vi "Main.vi"(0 "Temperature":dbl, 5 "Pressure":dbl, 7 "String 1":string, 9 "String 2":string, 11 "Error in":errorcluster) -> (15 "Error out":errorcluster)   [LabVIEW 2020, in "Menu.lvlib"]
doc: "This VI is just used to implement the run time menu feature where controls are enabled and disabled with the help of run time menu"
uses:
  Menu.lvlib
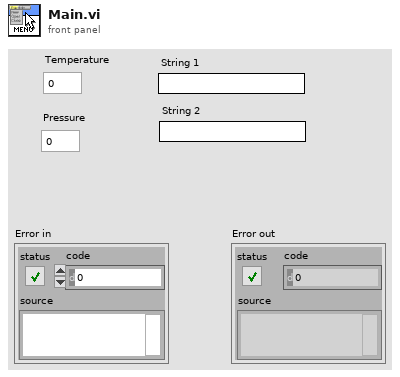
[diagram p1: front panel]
types:
  T1 = enum8{"Enabled", "Disabled", "Disabled and Grayed Out"}
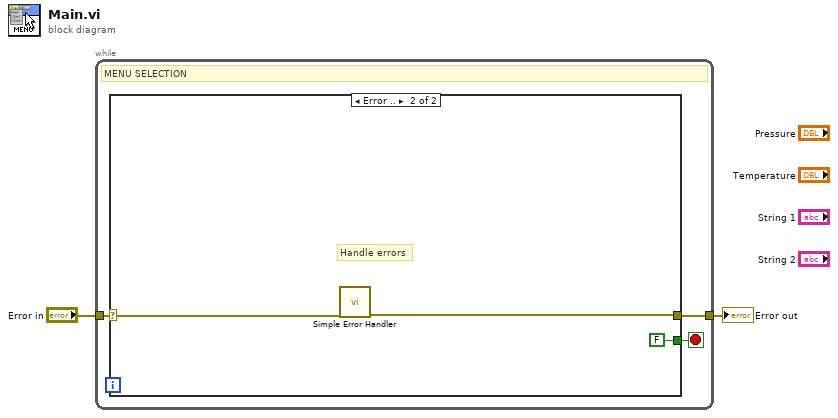
[diagram p0: block diagram]
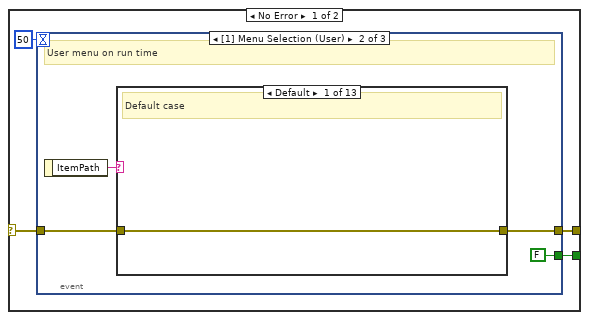
[diagram p2: hidden frame]
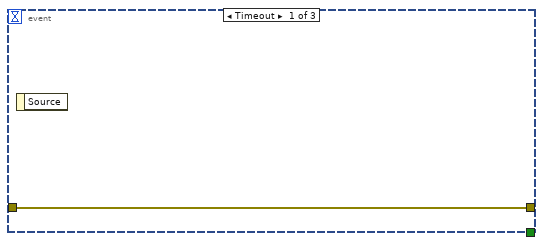
[diagram p3: hidden frame]
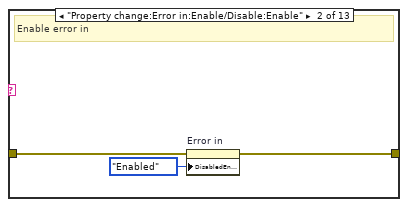
[diagram p4: hidden frame]
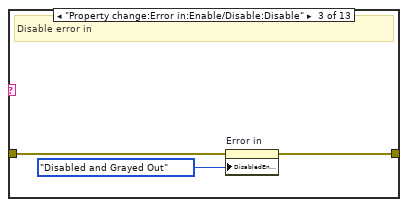
[diagram p5: hidden frame]
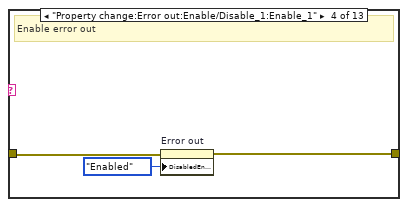
[diagram p6: hidden frame]
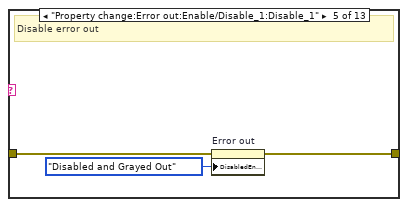
[diagram p7: hidden frame]
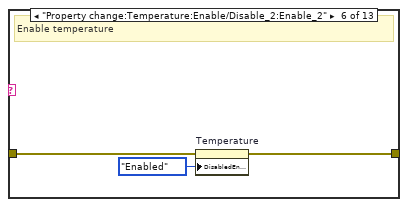
[diagram p8: hidden frame]
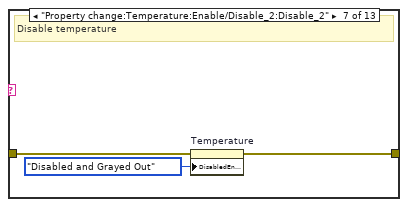
[diagram p9: hidden frame]
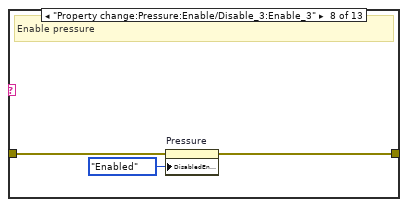
[diagram p10: hidden frame]
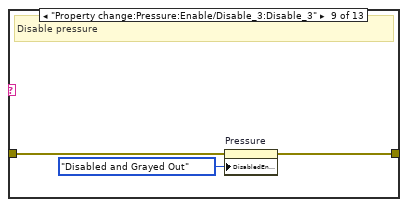
[diagram p11: hidden frame]
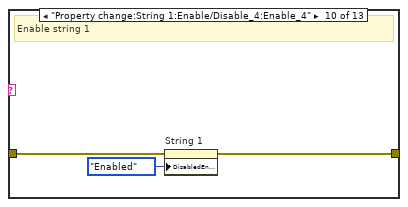
[diagram p12: hidden frame]
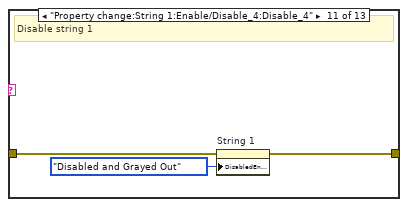
[diagram p13: hidden frame]
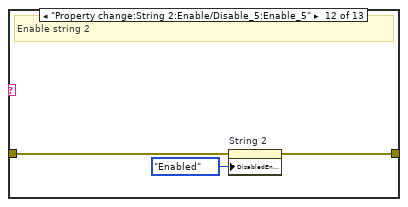
[diagram p14: hidden frame]
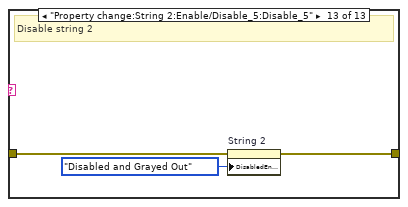
[diagram p15: hidden frame]
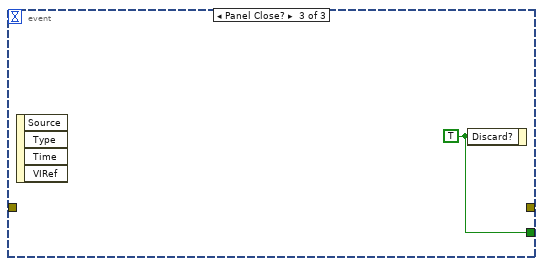
[diagram p16: hidden frame]
diagram:
  n1 = while {
    tunnel: "Error in" -> [w5]
    tunnel: [w4] -> w1
    stop <- w3 stop-if-true
    # "MENU SELECTION"
    n2 = case shown="Error .." w5 {
      selector: w5 -> [w8 w55]
      tunnel: [w7 w54] -> w4
      tunnel: [w6 FALSE ("Discard?")] -> w3
      frame No Error {
        n3 = event shown="[1] Menu Selection (User)" {
          selector: _ -> [_ _ _]
          dyn-events: _ -> [_ _ _]
          timeout: 50 -> [_ _ _]
          tunnel: w8 -> [w10 w12 _]
          tunnel: [w10 w11 _] -> w7
          tunnel: [_ FALSE ("Discard?") w52] -> w6
          event Timeout {
            n4 = event-data() -> ()  [unwired: 1 in, 1 out]
          }
          event Menu Selection (User) {
            # "User menu on run time"
            n5 = event-data() -> ("ItemPath"=w13:string)  [unwired: 1 in]
            n6 = case shown="Default" w13 {
              tunnel: w12 -> [w15 w18 w21 w23 w26 w30 w33 w36 w39 w42 w45 w48 w51]
              tunnel: [w15 w16 w20 w22 w25 w29 w32 w35 w38 w41 w44 w47 w50] -> w11
              frame Default {
                # "Default case"
              }
              frame "Property change:Error in:Enable/Disable:Enable" {
                # "Enable error in"
                n7 = property on="Error in" class="Clust (strict)"(error in=w18, "DisabledEnum"=T1."Enabled" ("Disabled")) -> (error out=w16:errorcluster)  [unwired: 1 in, 1 out]
              }
              frame "Property change:Error in:Enable/Disable:Disable" {
                # "Disable error in"
                n8 = property on="Error in" class="Clust (strict)"(error in=w21, "DisabledEnum"=T1."Disabled and Grayed Out" ("Disabled")) -> (error out=w20:errorcluster)  [unwired: 1 in, 1 out]
              }
              frame "Property change:Error out:Enable/Disable_1:Enable_1" {
                # "Enable error out"
                n9 = property on="Error out" class="Clust (strict)"(error in=w23, "DisabledEnum"=T1."Enabled" ("Disabled")) -> (error out=w22:errorcluster)  [unwired: 1 in, 1 out]
              }
              frame "Property change:Error out:Enable/Disable_1:Disable_1" {
                # "Disable error out"
                n10 = property on="Error out" class="Clust (strict)"(error in=w26, "DisabledEnum"=T1."Disabled and Grayed Out" ("Disabled")) -> (error out=w25:errorcluster)  [unwired: 1 in, 1 out]
              }
              frame "Property change:Temperature:Enable/Disable_2:Enable_2" {
                # "Enable temperature"
                n11 = property on="Temperature" class="DigNum (strict)"(error in=w30, "DisabledEnum"=T1."Enabled" ("Disabled")) -> (error out=w29:errorcluster)  [unwired: 1 in, 1 out]
              }
              frame "Property change:Temperature:Enable/Disable_2:Disable_2" {
                # "Disable temperature"
                n12 = property on="Temperature" class="DigNum (strict)"(error in=w33, "DisabledEnum"=T1."Disabled and Grayed Out" ("Disabled")) -> (error out=w32:errorcluster)  [unwired: 1 in, 1 out]
              }
              frame "Property change:Pressure:Enable/Disable_3:Enable_3" {
                # "Enable pressure"
                n13 = property on="Pressure" class="DigNum (strict)"(error in=w36, "DisabledEnum"=T1."Enabled" ("Disabled")) -> (error out=w35:errorcluster)  [unwired: 1 in, 1 out]
              }
              frame "Property change:Pressure:Enable/Disable_3:Disable_3" {
                # "Disable pressure"
                n14 = property on="Pressure" class="DigNum (strict)"(error in=w39, "DisabledEnum"=T1."Disabled and Grayed Out" ("Disabled")) -> (error out=w38:errorcluster)  [unwired: 1 in, 1 out]
              }
              frame "Property change:String 1:Enable/Disable_4:Enable_4" {
                # "Enable string 1"
                n15 = property on="String 1" class="Str"(error in=w42, "DisabledEnum"=T1."Enabled" ("Disabled")) -> (error out=w41:errorcluster)  [unwired: 1 in, 1 out]
              }
              frame "Property change:String 1:Enable/Disable_4:Disable_4" {
                # "Disable string 1"
                n16 = property on="String 1" class="Str"(error in=w45, "DisabledEnum"=T1."Disabled and Grayed Out" ("Disabled")) -> (error out=w44:errorcluster)  [unwired: 1 in, 1 out]
              }
              frame "Property change:String 2:Enable/Disable_5:Enable_5" {
                # "Enable string 2"
                n17 = property on="String 2" class="Str"(error in=w48, "DisabledEnum"=T1."Enabled" ("Disabled")) -> (error out=w47:errorcluster)  [unwired: 1 in, 1 out]
              }
              frame "Property change:String 2:Enable/Disable_5:Disable_5" {
                # "Disable string 2"
                n18 = property on="String 2" class="Str"(error in=w51, "DisabledEnum"=T1."Disabled and Grayed Out" ("Disabled")) -> (error out=w50:errorcluster)  [unwired: 1 in, 1 out]
              }
            }
          }
          event Panel Close? {
            w52 = TRUE ("Discard?")
            n19 = event-data() -> ()  [unwired: 1 in, 4 out]
            n20 = event-data("Discard?"=w52) -> ()  [unwired: 1 in, 1 out]
          }
        }
      }
      frame Error {
        # "Handle errors"
        n21 = call <vilib>:"Simple Error Handler.vi"("error in (no error)"=w55) -> ("error out"=w54:errorcluster)  [unwired: 4 in, 4 out]
      }
    }
  }
  "Error out" <- w1
